vi "Is DAC Enable.vi"(11 "channel":u8) -> (3 "function return":u8)   [LabVIEW 2021, in "vmmso.lvlib"]
doc: "DLL_API unsigned char WINAPI IsDACEnable(unsigned char channel);"
uses:
  vmmso.lvlib
  vmmso.dll
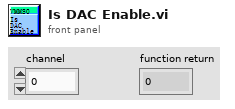
[diagram p1: front panel]
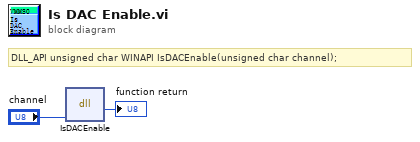
[diagram p0: block diagram]
diagram:
  # "DLL_API unsigned char WINAPI IsDACEnable(unsigned char channel);"
  n1 = dll-call lib="D:/labviewdemo/LabviewDemo 21/vmmso/vmmso.*" fn="IsDACEnable"("channel"="channel") -> (→"function return":u8)  [unwired: 4 in, 2 out]
